vi "Swerve_Main.vi"   [LabVIEW 2012]
uses:
  CLIB/CRef/Core/Master Types.ctl
  <vilib>/NXT/Block Support/NXT_OutputPort.ctl
  CLIB/CThread/Core/CThread Governor.vi
  CLIB/CThread/Core/CThread Termination Signal.vi
  CLIB/CRef/Interface/CRef Numeric.llb/CRef Get I32.vi
  Swerve_Slave.vi
  CLIB/CRef/LabelCore/CRefLabel Static Reference.vi
  CLIB/CRef/Interface/CRef Numeric.llb/CRef Set I32.vi
  <vilib>/NXT/Dual Mode Library/Waits/Wait_Num.vi
  <vilib>/NXT/NXTIO Xnodes/NXTIONodeSubVIs/NXTMoveMotors.vi
  CLIB/CThread/XNodes/initializernode/CThread Initializer.xnode
  CLIB/CRef/XNodes/labelnode/CRef Label Node.xnode
  <vilib>/NXT/NXTIO Xnodes/AddressXNode/NXTIOAddress.xnode
  <vilib>/NXT/NXTIO Xnodes/NXTIOXNode/NXTIO.xnode
  <vilib>/NXT/Subs/LVHSConnector.ctl
  <vilib>/NXT/LegoClasses/BrickReference/BrickReference.lvclass
  CLIB/CThread/CThread.lvlib
  CLIB/CRef/CRef.lvlib
types:
  T1 = typedef "LVHSConnector.ctl" = refnum<class "BrickReference.lvclass">
  T2 = typedef "NXT_OutputPort.ctl" = u8
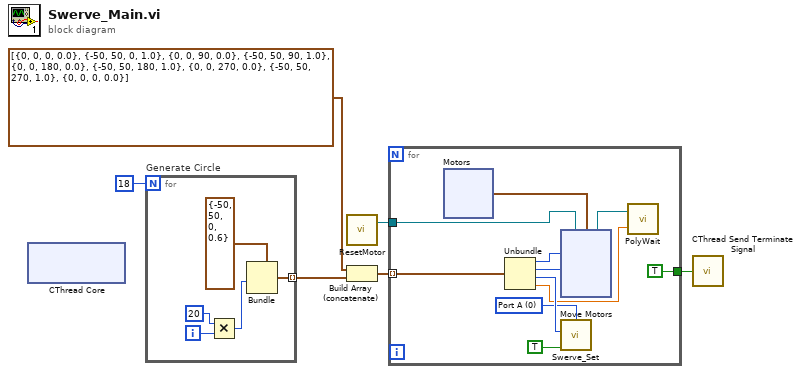
[diagram p0: block diagram]
diagram:
  n1 = xnode "CThread Core"() -> ()
  n2 = for "Generate Circle" {
    N: 18 -> [_]
    tunnel: [w10] -> w3 mode=indexing
    i -> [w7]
    n3 = Multiply(x=20, y=w7) -> (x*y=w8:i32)
    n4 = Bundle(cluster=cluster{i32, i32, i32, dbl} {-50, 50, 0, 0.6} ("Cluster"), w8) -> (w10:cluster{i32, i32, i32, dbl})  [unwired: 3 in]
  }
  n5 = call <vilib>:"ResetMotor.vi"() -> ("NXT/EV3"=w5:T1)  [unwired: 4 in]
  n6 = Build Array (concatenate)(cluster{i32, i32, i32, dbl}[] [{0, 0, 0, 0.0}, {-50, 50, 0, 1.0}, {0, 0, 90, 0.0}, {-50, 50, 90, 1.0}, {0, 0, 180, 0.0}, {-50, 50, 180, 1.0}, {0, 0, 270, 0.0}, {-50, 50, 270, 1.0}, {0, 0, 0, 0.0}], w3) -> (w2:cluster{i32, i32, i32, dbl}[])
  n7 = for {
    tunnel: w2 -> [w21] mode=indexing
    tunnel: [TRUE ("Terminate")] -> w6
    tunnel: w5 -> [w14]
    w12 = 0 items=["Port A", "Port B", "Port C", "Port D"] ("Port (Port A)")
    n8 = xnode "Motors"() -> ("Motor"=w22:cluster{"Port":T2, "Port":T2})
    n9 = Unbundle(w21) -> (w20:i32, w19:i32, w17:i32, w15:dbl)
    n10 = xnode "Move Motors"("Power/Speed 2"=w19, "Power/Speed 1"=w20, "Motors"=w22, "NXT/EV3"=w14) -> ("NXT/EV3"=w18:T1)
    n11 = call "Swerve_Set.vi"("Port (Port A)"=w12, "Intended Angle"=w17, "Wait? (T)"=TRUE ("Wait? (F)")) -> ()  [unwired: 6 in, 1 out]
    n12 = call-poly <vilib>:"PolyWait.vi"("Time (1 sec)"=w15, "NXT/EV3"=w18) -> ()  [unwired: 2 in, 1 out]
  }
  n13 = call "CThread Send Terminate Signal.vi"("Terminate"=w6) -> ()
